vi "Parse Control Label.vi"(11 "CtlRef":refnum<vi>) -> (2 "Value Name":string, 3 "Queue Name":string)   [LabVIEW 2018, in "Messaging.lvlib"]
uses:
  Messaging.lvlib
  <vilib>/regexp/Match Regular Expression.xnode
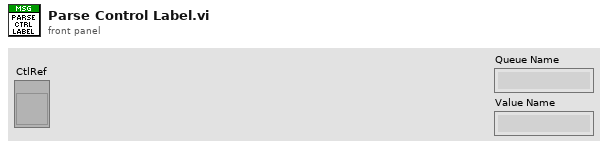
[diagram p1: front panel]
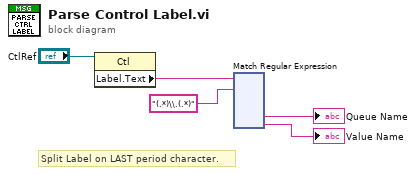
[diagram p0: block diagram]
diagram:
  # "Split Label on LAST period character."
  n1 = property class="Ctl"(reference="CtlRef") -> ("Label.Text"=w5:string)  [unwired: 1 in, 2 out]
  n2 = xnode "Match Regular Expression"("input string"=w5, "regular expression"="(.*)\\.(.*)") -> ("submatch 1"=→"Queue Name":string, "submatch 2"=→"Value Name":string)  [unwired: 4 in, 5 out]
